vi "substates.vi"() -> (0 "Loop 3: Tote Pistons":T1, 1 "Loop 2: Container Arm":T2, 2 "Loop 1: Lift":T2, 3 "Loop 0: Drive":T2)   [LabVIEW 2014]
uses:
  Type Defs/subStates.ctl
  Type Defs/singleUseSubstate.ctl
  <vilib>/Rock Robotics/Network Tables/NT Read Numeric Array.vi
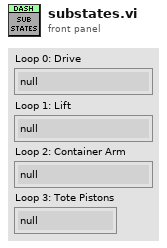
[diagram p1: front panel]
types:
  T1 = typedef "singleUseSubstate.ctl" = enum16{"null", "wait", "extend", "retract", "end"}
  T2 = typedef "subStates.ctl" = enum16{"null", "wait", "driver control", "auto", "manual override", "hold position", "rotate", "test", "end"}
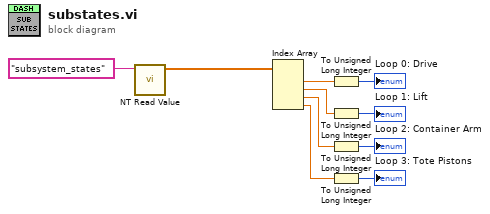
[diagram p0: block diagram]
diagram:
  n1 = call-poly <vilib>:"NT Read Value.vi"("Name"="subsystem_states") -> ("Numeric Array"=w9:dbl[])  [unwired: 9 in, 1 out]
  n2 = Index Array(array=w9) -> (element #1=w8:dbl, element #2=w5:dbl, element #3=w3:dbl, element #4=w1:dbl)  [unwired: 4 in]
  n3 = To Unsigned Long Integer(number=w8) -> (unsigned 32bit integer=→"Loop 0: Drive":u32)
  n4 = To Unsigned Long Integer(number=w5) -> (unsigned 32bit integer=→"Loop 1: Lift":u32)
  n5 = To Unsigned Long Integer(number=w3) -> (unsigned 32bit integer=→"Loop 2: Container Arm":u32)
  n6 = To Unsigned Long Integer(number=w1) -> (unsigned 32bit integer=→"Loop 3: Tote Pistons":u32)
